vi "Begin.vi"(8 "error in":errorcluster) -> (0 "error out":errorcluster)   [LabVIEW 2019]
doc: "Called before other user functions, this VI is expected to open initial I/O refnums, load in file data, and do all program initialization. Notice that the <B>error out</B> terminal is simply used for data flow. Wiring it to other structures or subVIs ensures that this VI runs first."
uses:
  <vilib>/Rock Robotics/WPI/DriverStation/WPI_DriverStationRobotMode2.ctl
  <vilib>/Rock Robotics/WPI/Joystick/WPI_JoystickDeviceEnum.ctl
  Subsystems/Drive/Drive_Cluster.ctl
  Subsystems/Drive/Drive_Control_States.ctl
  Subsystems/Drive/Drive_Orientation_States.ctl
  <vilib>/Rock Robotics/WPI/ThirdParty/Phoenix-LabVIEW/Motor Controller/Controls/CTRE_Phoenix_MotorControl_TalonFXInvertType.ctl
  <vilib>/Rock Robotics/WPI/ThirdParty/Phoenix-LabVIEW/Motor Controller/Controls/CTRE_Phoenix_MotorControl_NeutralMode.ctl
  Robot Global Data.vi
  Globals/Drive_Globals.vi
  <vilib>/Rock Robotics/WPI/ThirdParty/Phoenix-LabVIEW/Pigeon IMU/CTRE_PigeonIMU_Open_TalonSRX.vi
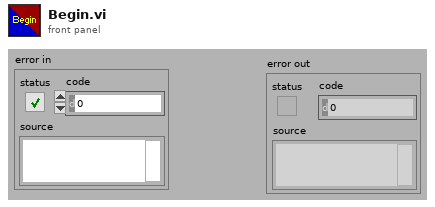
[diagram p1: front panel]
types:
  T1 = typedef "CTRE_Phoenix_MotorControl_NeutralMode.ctl" = enum8{"EEPROMSetting", "Override to Coast", "Override to Brake"}
  T2 = typedef "CTRE_Phoenix_MotorControl_TalonFXInvertType.ctl" = enum16{"Counter-Clockwise", "Clockwise"}
  T3 = typedef "Drive_Cluster.ctl" = cluster{"Control_State":T4, "Vertical_Throttle":dbl, "Lateral_Throttle":dbl, "Rotational_Throttle":dbl, "Strafe_In_Deadband":bool, "Rotation_In_Deadband":bool, "Orientation_State":T5}
  T4 = typedef "Drive_Control_States.ctl" = enum16{"Manual_Control", ""}
  T5 = typedef "Drive_Orientation_States.ctl" = enum16{"Robot-Oriented", "Field-Oriented"}
  T6 = typedef "WPI_JoystickDeviceEnum.ctl" = enum16{"USB 0", "USB 1", "USB 2", "USB 3", "USB 4", "USB 5"}
  T7 = typedef "WPI_DriverStationRobotMode2.ctl" = enum16{"Autonomous Disabled", "Autonomous Enabled", "Teleop Disabled", "Teleop Enabled", "Disconnected", "Finish", "Test Disabled", "Test Enabled", "Emergency Stopped"}
  T8 = typedef "WPI_MotorControlDeviceRef.ctl" = cluster{"DeviceStatus":errorcluster, "Type":T9, "PWM":cluster{"PWM Channel":T10, "DeadBand":T11}, "CAN":cluster{"Device Number":u8, "SetOutput VI Ref":variant, "GetOutput VI Ref":variant, "Enable VI Ref":variant, "Disable VI Ref":variant, "Data":variant}, "Invert":bool, "DIO PWM":cluster{"PWM \"Enable\" Channel":T10, "DIOChannel":T12, "PWM Rate":dbl}}
  T9 = typedef "WPI_MotorControlType.ctl" = enum16{"PWM", "CAN", "DIO PWM"}
  T10 = typedef "FPGA_DIOPWMChannel.ctl" = enum8{"PWM 0", "PWM 1", "PWM 2", "PWM 3", "PWM 4", "PWM 5", "PWM 6", "PWM 7", "PWM 8", "PWM 9", "PWM MXP 0", "PWM MXP 1", "PWM MXP 2", "PWM MXP 3", "PWM MXP 4", "PWM MXP 5", "PWM MXP 6", "PWM MXP 7", "PWM MXP 8", "PWM MXP 9", "Invalid"}
  T11 = typedef "WPI_PWMDeadband.ctl" = cluster{"Name":string, "maxPositivePwm":i32, "minPositivePwm":i32, "centerPwm":i32, "maxNegativePwm":i32, "minNegativePwm":i32, "angularRange":u16}
  T12 = typedef "FPGA_DIOChannel.ctl" = enum8{"DIO 0", "DIO 1", "DIO 2", "DIO 3", "DIO 4", "DIO 5", "DIO 6", "DIO 7", "DIO 8", "DIO 9", "DIO MXP 0", "DIO MXP 1", "DIO MXP 2", "DIO MXP 3", "DIO MXP 4", "DIO MXP 5", "DIO MXP 6", "DIO MXP 7", "DIO MXP 8", "DIO MXP 9", "DIO MXP 10", "DIO MXP 11", "DIO MXP 12", "DIO MXP 13", "DIO MXP 14", "DIO MXP 15", "SPI Port CS1", "SPI Port CS2", "SPI Port CS3", "SPI Port MISO", "SPI Port MOSI", "Invalid"}
  T13 = typedef "WPI_JoystickDevRef.ctl" = cluster{"Device":T6}
  T14 = typedef "CTRE_PigeonIMU_DeviceRef.ctl" = cluster{"DeviceStatus":errorcluster, "Device Number":u8, "Type":T15, "Device ID":u32, "Handle":u64, "UsageFrame":u32, "Library Path":path}
  T15 = typedef "CTRE_PigeonIMU_ConnectionType.ctl" = u32
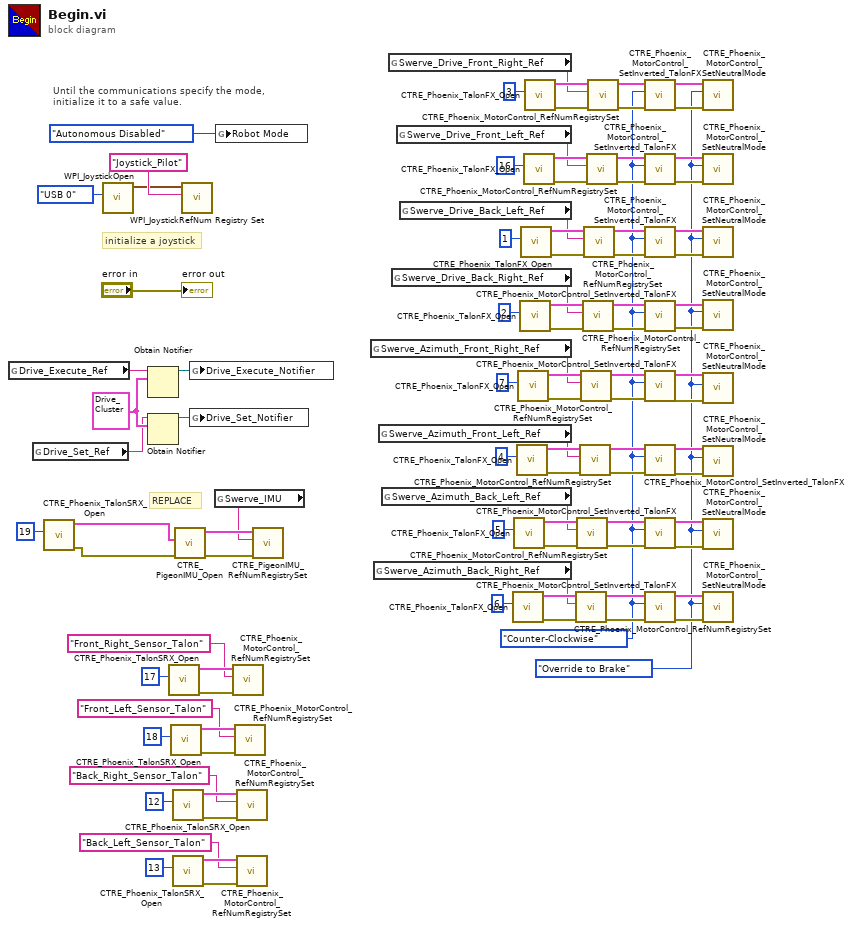
[diagram p0: block diagram]
diagram:
  w4 = CTRE_Phoenix_MotorControl_NeutralMode."Override to Brake" ("Motor Control Neutral Mode")
  w38 = CTRE_Phoenix_MotorControl_TalonFXInvertType."Counter-Clockwise" ("Invert Type")
  w93 = T3 {"Control_State"=enum."Manual_Control", "Vertical_Throttle"=0.0, "Lateral_Throttle"=0.0, "Rotational_Throttle"=0.0, "Strafe_In_Deadband"=FALSE, "Rotation_In_Deadband"=FALSE, "Orientation_State"=enum."Robot-Oriented"}
  # "REPLACE"
  # "initialize a joystick"
  # "Until the communications specify the mode,\ninitialize it to a safe value."
  n1 = global read "Drive_Globals.vi" "Drive_Execute_Ref"() -> (w92:string)
  n2 = global read "Drive_Globals.vi" "Drive_Set_Ref"() -> (w91:string)
  n3 = call <vilib>:"CTRE_Phoenix_TalonSRX_Open.vi"("Device Number"=u8 19) -> ("error out"=w1:errorcluster, "CAN Talon SRX Ref"=w2:T8)  [unwired: 9 in]
  n4 = call <vilib>:"WPI_JoystickOpen.vi"("JoystickDevice"=WPI_JoystickDeviceEnum."USB 0") -> ("JoystickDevRef"=w96:T13)  [unwired: 10 in]
  n5 = Obtain Notifier(name (unnamed)=w92, notification data type=w93) -> (notifier out=w90:refnum<notifier>)  [unwired: 2 in, 2 out]
  n6 = Obtain Notifier(name (unnamed)=w91, notification data type=w93) -> (notifier out=w89:refnum<notifier>)  [unwired: 2 in, 2 out]
  n7 = call <vilib>:"CTRE_Phoenix_TalonSRX_Open.vi"("Device Number"=u8 17) -> ("error out"=w35:errorcluster, "CAN Talon SRX Ref"=w36:T8)  [unwired: 9 in]
  n8 = call <vilib>:"CTRE_Phoenix_TalonSRX_Open.vi"("Device Number"=u8 18) -> ("error out"=w34:errorcluster, "CAN Talon SRX Ref"=w33:T8)  [unwired: 9 in]
  n9 = call <vilib>:"CTRE_Phoenix_TalonSRX_Open.vi"("Device Number"=u8 12) -> ("error out"=w31:errorcluster, "CAN Talon SRX Ref"=w32:T8)  [unwired: 9 in]
  n10 = call <vilib>:"CTRE_Phoenix_TalonSRX_Open.vi"("Device Number"=u8 13) -> ("error out"=w30:errorcluster, "CAN Talon SRX Ref"=w29:T8)  [unwired: 9 in]
  n11 = call-poly <vilib>:"CTRE_PigeonIMU_Open.vi"("error in"=w1, "CAN Talon SRX Ref"=w2) -> ("error out"=w87:errorcluster, "PigeonIMUDevRef"=w88:T14)  [unwired: 8 in]
  n12 = call <vilib>:"WPI_JoystickRefNum Registry Set.vi"("refnum name"="Joystick_Pilot", "JoystickDevRef"=w96) -> ()  [unwired: 8 in, 2 out]
  n13 = global write "Drive_Globals.vi" "Drive_Execute_Notifier"(w90) -> ()
  n14 = global write "Drive_Globals.vi" "Drive_Set_Notifier"(w89) -> ()
  n15 = global read "Drive_Globals.vi" "Swerve_IMU"() -> (w37:string)
  n16 = global write "Robot Global Data.vi" "Robot Mode"(WPI_DriverStationRobotMode2."Autonomous Disabled" ("Robot Mode")) -> ()
  n17 = call <vilib>:"CTRE_Phoenix_MotorControl_RefNumRegistrySet.vi"("error in (no error)"=w35, "refnum name"="Front_Right_Sensor_Talon", "PhoenixMotorControlDevRef"=w36) -> ()  [unwired: 7 in, 2 out]
  n18 = call <vilib>:"CTRE_Phoenix_MotorControl_RefNumRegistrySet.vi"("error in (no error)"=w34, "refnum name"="Front_Left_Sensor_Talon", "PhoenixMotorControlDevRef"=w33) -> ()  [unwired: 7 in, 2 out]
  n19 = call <vilib>:"CTRE_Phoenix_MotorControl_RefNumRegistrySet.vi"("error in (no error)"=w31, "refnum name"="Back_Right_Sensor_Talon", "PhoenixMotorControlDevRef"=w32) -> ()  [unwired: 7 in, 2 out]
  n20 = call <vilib>:"CTRE_Phoenix_MotorControl_RefNumRegistrySet.vi"("error in (no error)"=w30, "refnum name"="Back_Left_Sensor_Talon", "PhoenixMotorControlDevRef"=w29) -> ()  [unwired: 7 in, 2 out]
  n21 = call <vilib>:"CTRE_PigeonIMU_RefNumRegistrySet.vi"("error in (no error)"=w87, "refnum name"=w37, "PigeonIMUDevRef"=w88) -> ()  [unwired: 7 in, 2 out]
  n22 = global read "Drive_Globals.vi" "Swerve_Azimuth_Front_Right_Ref"() -> (w42:string)
  n23 = global read "Drive_Globals.vi" "Swerve_Azimuth_Back_Right_Ref"() -> (w39:string)
  n24 = global read "Drive_Globals.vi" "Swerve_Azimuth_Front_Left_Ref"() -> (w41:string)
  n25 = global read "Drive_Globals.vi" "Swerve_Azimuth_Back_Left_Ref"() -> (w40:string)
  n26 = global read "Drive_Globals.vi" "Swerve_Drive_Front_Right_Ref"() -> (w46:string)
  n27 = global read "Drive_Globals.vi" "Swerve_Drive_Back_Right_Ref"() -> (w43:string)
  n28 = global read "Drive_Globals.vi" "Swerve_Drive_Front_Left_Ref"() -> (w45:string)
  n29 = global read "Drive_Globals.vi" "Swerve_Drive_Back_Left_Ref"() -> (w44:string)
  n30 = call <vilib>:"CTRE_Phoenix_TalonFX_Open.vi"("Device Number"=u8 6) -> ("error out"=w60:errorcluster, "CAN Talon SRX Ref"=w57:T8)  [unwired: 9 in]
  n31 = call <vilib>:"CTRE_Phoenix_TalonFX_Open.vi"("Device Number"=u8 5) -> ("error out"=w63:errorcluster, "CAN Talon SRX Ref"=w66:T8)  [unwired: 9 in]
  n32 = call <vilib>:"CTRE_Phoenix_TalonFX_Open.vi"("Device Number"=u8 4) -> ("error out"=w53:errorcluster, "CAN Talon SRX Ref"=w56:T8)  [unwired: 9 in]
  n33 = call <vilib>:"CTRE_Phoenix_TalonFX_Open.vi"("Device Number"=u8 7) -> ("error out"=w50:errorcluster, "CAN Talon SRX Ref"=w47:T8)  [unwired: 9 in]
  n34 = call <vilib>:"CTRE_Phoenix_TalonFX_Open.vi"("Device Number"=u8 2) -> ("error out"=w73:errorcluster, "CAN Talon SRX Ref"=w76:T8)  [unwired: 9 in]
  n35 = call <vilib>:"CTRE_Phoenix_TalonFX_Open.vi"("Device Number"=u8 1) -> ("error out"=w70:errorcluster, "CAN Talon SRX Ref"=w67:T8)  [unwired: 9 in]
  n36 = call <vilib>:"CTRE_Phoenix_TalonFX_Open.vi"("Device Number"=u8 16) -> ("error out"=w80:errorcluster, "CAN Talon SRX Ref"=w77:T8)  [unwired: 9 in]
  n37 = call <vilib>:"CTRE_Phoenix_TalonFX_Open.vi"("Device Number"=u8 3) -> ("error out"=w83:errorcluster, "CAN Talon SRX Ref"=w86:T8)  [unwired: 9 in]
  n38 = call <vilib>:"CTRE_Phoenix_MotorControl_RefNumRegistrySet.vi"("error in (no error)"=w60, "refnum name"=w39, "PhoenixMotorControlDevRef"=w57) -> ("error out"=w59:errorcluster, "PhoenixMotorControlDevRef"=w58:T8)  [unwired: 7 in]
  n39 = call <vilib>:"CTRE_Phoenix_MotorControl_RefNumRegistrySet.vi"("error in (no error)"=w63, "refnum name"=w40, "PhoenixMotorControlDevRef"=w66) -> ("error out"=w64:errorcluster, "PhoenixMotorControlDevRef"=w65:T8)  [unwired: 7 in]
  n40 = call <vilib>:"CTRE_Phoenix_MotorControl_RefNumRegistrySet.vi"("error in (no error)"=w53, "refnum name"=w41, "PhoenixMotorControlDevRef"=w56) -> ("error out"=w54:errorcluster, "PhoenixMotorControlDevRef"=w55:T8)  [unwired: 7 in]
  n41 = call <vilib>:"CTRE_Phoenix_MotorControl_RefNumRegistrySet.vi"("error in (no error)"=w50, "refnum name"=w42, "PhoenixMotorControlDevRef"=w47) -> ("error out"=w49:errorcluster, "PhoenixMotorControlDevRef"=w48:T8)  [unwired: 7 in]
  n42 = call <vilib>:"CTRE_Phoenix_MotorControl_RefNumRegistrySet.vi"("error in (no error)"=w73, "refnum name"=w43, "PhoenixMotorControlDevRef"=w76) -> ("error out"=w74:errorcluster, "PhoenixMotorControlDevRef"=w75:T8)  [unwired: 7 in]
  n43 = call <vilib>:"CTRE_Phoenix_MotorControl_RefNumRegistrySet.vi"("error in (no error)"=w70, "refnum name"=w44, "PhoenixMotorControlDevRef"=w67) -> ("error out"=w69:errorcluster, "PhoenixMotorControlDevRef"=w68:T8)  [unwired: 7 in]
  n44 = call <vilib>:"CTRE_Phoenix_MotorControl_RefNumRegistrySet.vi"("error in (no error)"=w80, "refnum name"=w45, "PhoenixMotorControlDevRef"=w77) -> ("error out"=w79:errorcluster, "PhoenixMotorControlDevRef"=w78:T8)  [unwired: 7 in]
  n45 = call <vilib>:"CTRE_Phoenix_MotorControl_RefNumRegistrySet.vi"("error in (no error)"=w83, "refnum name"=w46, "PhoenixMotorControlDevRef"=w86) -> ("error out"=w84:errorcluster, "PhoenixMotorControlDevRef"=w85:T8)  [unwired: 7 in]
  n46 = call <vilib>:"CTRE_Phoenix_MotorControl_SetInverted_TalonFX.vi"("error in (no error)"=w84, "Invert Type"=w38, "PhoenixMotorControlDevRef"=w85) -> ("error out"=w17:errorcluster, "PhoenixMotorControlDevRef"=w18:T8)  [unwired: 7 in]
  n47 = call <vilib>:"CTRE_Phoenix_MotorControl_SetInverted_TalonFX.vi"("error in (no error)"=w79, "Invert Type"=w38, "PhoenixMotorControlDevRef"=w78) -> ("error out"=w15:errorcluster, "PhoenixMotorControlDevRef"=w16:T8)  [unwired: 7 in]
  n48 = call <vilib>:"CTRE_Phoenix_MotorControl_SetInverted_TalonFX.vi"("error in (no error)"=w69, "Invert Type"=w38, "PhoenixMotorControlDevRef"=w68) -> ("error out"=w13:errorcluster, "PhoenixMotorControlDevRef"=w14:T8)  [unwired: 7 in]
  n49 = call <vilib>:"CTRE_Phoenix_MotorControl_SetInverted_TalonFX.vi"("error in (no error)"=w74, "Invert Type"=w38, "PhoenixMotorControlDevRef"=w75) -> ("error out"=w11:errorcluster, "PhoenixMotorControlDevRef"=w12:T8)  [unwired: 7 in]
  n50 = call <vilib>:"CTRE_Phoenix_MotorControl_SetInverted_TalonFX.vi"("error in (no error)"=w49, "Invert Type"=w38, "PhoenixMotorControlDevRef"=w48) -> ("error out"=w9:errorcluster, "PhoenixMotorControlDevRef"=w10:T8)  [unwired: 7 in]
  n51 = call <vilib>:"CTRE_Phoenix_MotorControl_SetInverted_TalonFX.vi"("error in (no error)"=w54, "Invert Type"=w38, "PhoenixMotorControlDevRef"=w55) -> ("error out"=w7:errorcluster, "PhoenixMotorControlDevRef"=w8:T8)  [unwired: 7 in]
  n52 = call <vilib>:"CTRE_Phoenix_MotorControl_SetInverted_TalonFX.vi"("error in (no error)"=w64, "Invert Type"=w38, "PhoenixMotorControlDevRef"=w65) -> ("error out"=w5:errorcluster, "PhoenixMotorControlDevRef"=w6:T8)  [unwired: 7 in]
  n53 = call <vilib>:"CTRE_Phoenix_MotorControl_SetInverted_TalonFX.vi"("error in (no error)"=w59, "Invert Type"=w38, "PhoenixMotorControlDevRef"=w58) -> ("error out"=w19:errorcluster, "PhoenixMotorControlDevRef"=w20:T8)  [unwired: 7 in]
  n54 = call <vilib>:"CTRE_Phoenix_MotorControl_SetNeutralMode.vi"("error in (no error)"=w17, "Motor Control Neutral Mode"=w4, "PhoenixMotorControlDevRef"=w18) -> ()  [unwired: 7 in, 2 out]
  n55 = call <vilib>:"CTRE_Phoenix_MotorControl_SetNeutralMode.vi"("error in (no error)"=w15, "Motor Control Neutral Mode"=w4, "PhoenixMotorControlDevRef"=w16) -> ()  [unwired: 7 in, 2 out]
  n56 = call <vilib>:"CTRE_Phoenix_MotorControl_SetNeutralMode.vi"("error in (no error)"=w13, "Motor Control Neutral Mode"=w4, "PhoenixMotorControlDevRef"=w14) -> ()  [unwired: 7 in, 2 out]
  n57 = call <vilib>:"CTRE_Phoenix_MotorControl_SetNeutralMode.vi"("error in (no error)"=w11, "Motor Control Neutral Mode"=w4, "PhoenixMotorControlDevRef"=w12) -> ()  [unwired: 7 in, 2 out]
  n58 = call <vilib>:"CTRE_Phoenix_MotorControl_SetNeutralMode.vi"("error in (no error)"=w9, "Motor Control Neutral Mode"=w4, "PhoenixMotorControlDevRef"=w10) -> ()  [unwired: 7 in, 2 out]
  n59 = call <vilib>:"CTRE_Phoenix_MotorControl_SetNeutralMode.vi"("error in (no error)"=w7, "Motor Control Neutral Mode"=w4, "PhoenixMotorControlDevRef"=w8) -> ()  [unwired: 7 in, 2 out]
  n60 = call <vilib>:"CTRE_Phoenix_MotorControl_SetNeutralMode.vi"("error in (no error)"=w5, "Motor Control Neutral Mode"=w4, "PhoenixMotorControlDevRef"=w6) -> ()  [unwired: 7 in, 2 out]
  n61 = call <vilib>:"CTRE_Phoenix_MotorControl_SetNeutralMode.vi"("error in (no error)"=w19, "Motor Control Neutral Mode"=w4, "PhoenixMotorControlDevRef"=w20) -> ()  [unwired: 7 in, 2 out]
  "error out" <- "error in"
